vi "Excel - Macro.vi"() -> ()   [LabVIEW 2023]
doc: "This example demonstrates how to run a macro on an Excel worksheet to display the worksheet data in an Excel graph."
panel:
  in  "Macro Name":string="GraphData"
  # "Overview: Demonstrates how to run a macro on an Excel worksheet to display the worksheet data in an Excel graph.\nRequirements: Windows with Microsoft Excel\nInstructions:\nRun the VI."
  # "See the block diagram for more information on how to execute macros in Microsoft Excel."
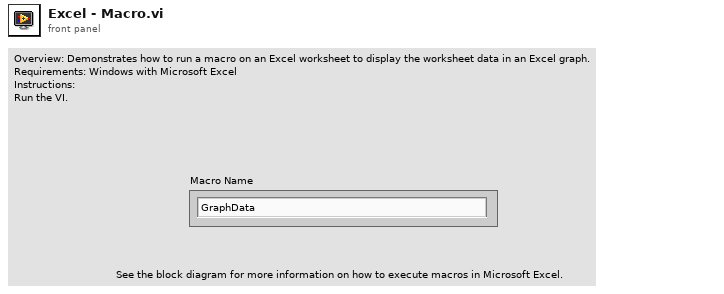
[diagram p1: front panel]
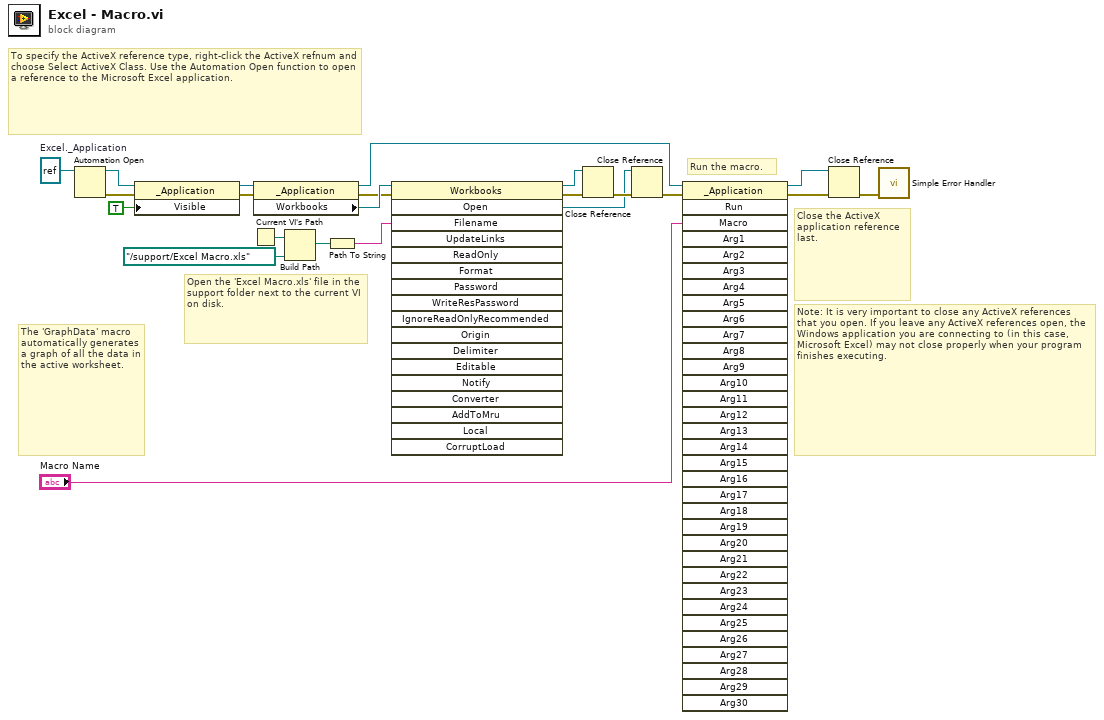
[diagram p0: block diagram]
diagram:
  w13 = refnum<k7> refnum  # Excel._Application
  # "Note: It is very important to close any ActiveX references that you open. If you leave any ActiveX references open, the Windows application you are connecting to (in this case, Microsoft Excel) may not close properly when your program finishes executing."
  # "Run the macro."
  # "The 'GraphData' macro  automatically generates a graph of all the data in the active worksheet."
  # "Close the ActiveX application reference last."
  # "Open the 'Excel Macro.xls' file in the support folder next to the current VI on disk."
  # "To specify the ActiveX reference type, right-click the ActiveX refnum and choose Select ActiveX Class. Use the Automation Open function to open a reference to the Microsoft Excel application."
  n1 = Automation Open(Automation Refnum=w13) -> (Automation Refnum=w14:refnum<k7>, error out=w15:errorcluster)  [unwired: 1 in, 2 out]
  n2 = property class="_Application"(reference=w14, error in=w15, "Visible"=TRUE) -> (reference out=w5:refnum<k7>, error out=w7:errorcluster)
  n3 = Current VI's Path() -> (path=w16:path)
  n4 = property class="_Application"(reference=w5, error in=w7) -> (reference out=w4:refnum<k7>, error out=w11:errorcluster, "Workbooks"=w12:refnum<k7>)
  n5 = Build Path(base path=w16, name or relative path=path "../support/Excel Macro.xls" ("Workbook Name")) -> (appended path=w18:path)
  n6 = Path To String(path=w18) -> (string=w8:string)
  n7 = invoke class="Workbooks" method="Open"(reference=w12, error in=w11, "Filename"=w8) -> (reference out=w9:refnum<k7>, error out=w10:errorcluster, "Open"=w1:refnum<k7>)  [unwired: 15 in, 15 out]
  n8 = Close Reference(reference=w9, error in (no error)=w10) -> (error out=w3:errorcluster)
  n9 = Close Reference(reference=w1, error in (no error)=w3) -> (error out=w2:errorcluster)
  n10 = invoke class="_Application" method="Run"(reference=w4, error in=w2, "Macro"="Macro Name") -> (reference out=w17:refnum<k7>, error out=w20:errorcluster)  [unwired: 31 in, 32 out]
  n11 = Close Reference(reference=w17, error in (no error)=w20) -> (error out=w22:errorcluster)
  n12 = call <vilib>:"Simple Error Handler.vi"("error in (no error)"=w22) -> ()  [unwired: 4 in, 5 out]
